vi "Check Multiple Uses same HW Configuration File.vi"(8 "error in (no error)":errorcluster, 11 "Item Ref in":T1 format="%.0x") -> (0 "error out":errorcluster)   [LabVIEW 2019, in "Ballard Arinc-429 System Explorer.lvlib"]
uses:
  Ballard Arinc-429 System Explorer.lvlib
  <vilib>/NI VeriStand/Custom Device API/Custom Device Item Ref.ctl
  Shared/Controls and Global/Global.vi
  <vilib>/NI VeriStand/Custom Device Tools/Custom Device Utility Library/NI VeriStand - Search for All Items by GUID.vi
  <vilib>/NI VeriStand/Custom Device API/Get Item Property (Path).vi
  <userlib>/_OpenG.lib/md5/md5.llb/MD5 Message Digest (Binary String)__ogtk.vi
  <userlib>/_OpenG.lib/array/array.llb/Remove Duplicates from 1D Array (String)__ogtk.vi
  <vilib>/NI VeriStand/Custom Device API/Custom Device API.lvlib
  <vilib>/NI VeriStand/Custom Device Tools/Custom Device Utility Library/Custom Device Utility Library.lvlib
  Shared/Ballard Arinc-429 Shared.lvlib
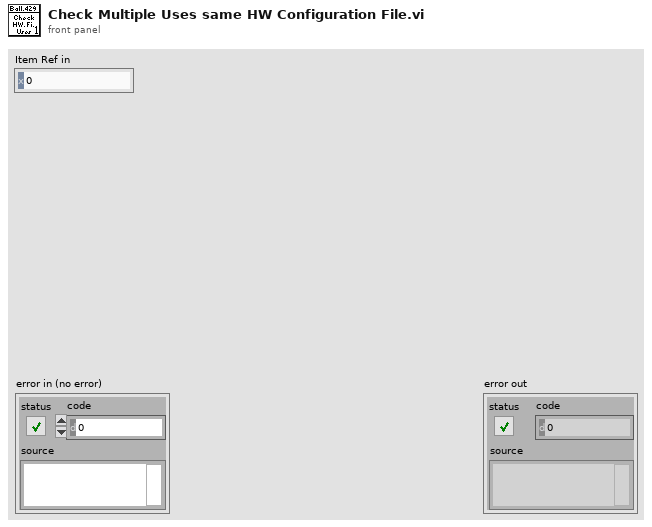
[diagram p1: front panel]
types:
  T1 = typedef "Custom Device API.lvlib/Custom Device Item Ref.ctl" = u64
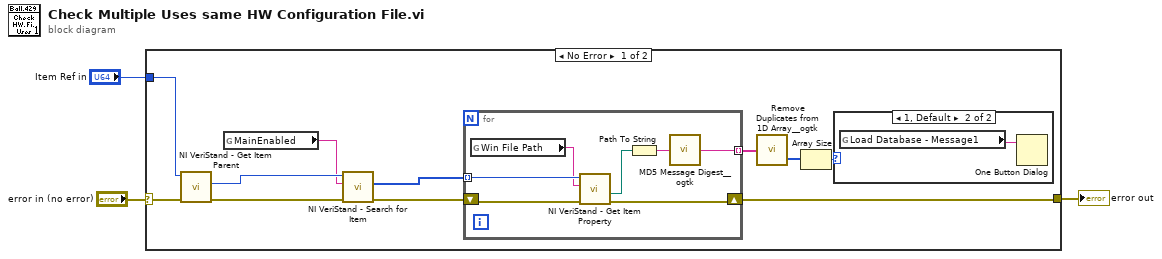
[diagram p0: block diagram]
diagram:
  n1 = case shown="No Error" "error in (no error)" {
    selector: "error in (no error)" -> [w14 w23]
    tunnel: [w5 w23] -> w2
    tunnel: "Item Ref in" -> [w13 _]
    frame No Error {
      n2 = call <vilib>:"NI VeriStand - Get Item Parent.vi"("error in (no error)"=w14, "Item Ref in"=w13) -> ("error out"=w12:errorcluster, "Parent Ref"=w11:T1)  [unwired: 6 in, 2 out]
      n3 = global read "Global.vi" "MainEnabled"() -> (w10:string)
      n4 = call-poly <vilib>:"NI VeriStand - Search for Item.vi"("error in"=w12, "Item GUID"=w10, "Section Ref in"=w11) -> ("error out"=w8:errorcluster, "Item Refs"=w9:T1[])  [unwired: 5 in, 2 out]
      n5 = for {
        tunnel: w9 -> [w22] mode=indexing
        shift-right: [w18] -> w5
        shift-left: w8 -> [w21]
        tunnel: [w16] -> w7 mode=indexing
        n6 = global read "Global.vi" "Win File Path"() -> (w20:string)
        n7 = call-poly <vilib>:"NI VeriStand - Get Item Property.vi"("error in (no error)"=w21, "Property Name"=w20, "Item Ref in"=w22) -> ("error out"=w18:errorcluster, "Value"=w19:path)  [unwired: 5 in, 2 out]
        n8 = Path To String(path=w19) -> (string=w17:string)
        n9 = call-poly <userlib>:"MD5 Message Digest__ogtk.vi"("Message"=w17) -> ("MD5 Message Digest"=w16:string)
      }
      n10 = call-poly <userlib>:"Remove Duplicates from 1D Array__ogtk.vi"("Input Array"=w7) -> ("indices of removed elements"=w6:i32[])  [unwired: 1 out]
      n11 = Array Size(array=w6) -> (size(s)=w4:i32)
      n12 = case shown="1, Default" w4 {
        frame 0 {
        }
        frame 1, Default {
          n13 = global read "Global.vi" "Load Database - Message1"() -> (w15:string)
          n14 = One Button Dialog(message=w15) -> ()  [unwired: 1 in, 1 out]
        }
      }
    }
    frame Error {
    }
  }
  "error out" <- w2
